vi "lab_abcd.vi"() -> ()   [LabVIEW 2023]
panel:
  out "x .or. y?":bool
  in  "d_in":bool=TRUE
  in  "b_in":bool=TRUE
  in  "c_in":bool
  in  "a_in":bool
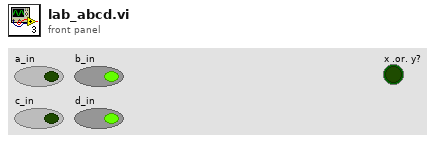
[diagram p1: front panel]
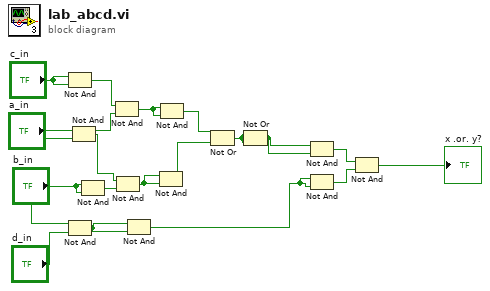
[diagram p0: block diagram]
diagram:
  n1 = Not And(1:"c_in", 2:"c_in") -> (0:w17:bool)
  n2 = Not And(1:"d_in", 2:"b_in") -> (0:w12:bool)
  n3 = Not And(1:"a_in", 2:"a_in") -> (0:w10:bool)
  n4 = Not And(1:"b_in", 2:"b_in") -> (0:w9:bool)
  n5 = Not And(1:"a_in", 2:w17) -> (0:w15:bool)
  n6 = Not And(1:w9, 2:w10) -> (0:w11:bool)
  n7 = Not And(1:w12, 2:w12) -> (0:w4:bool)
  n8 = Not And(1:w11, 2:w11) -> (0:w7:bool)
  n9 = Not And(1:w15, 2:w15) -> (0:w6:bool)
  n10 = Not Or(1:w7, 2:w6) -> (0:w8:bool)
  n11 = Not Or(1:w8, 2:w8) -> (0:w5:bool)
  n12 = Not And(1:w5, 2:w5) -> (0:w3:bool)
  n13 = Not And(1:w4, 2:w4) -> (0:w2:bool)
  n14 = Not And(1:w2, 2:w3) -> (0:→"x .or. y?":bool)
